vi "0 - Shooting v2.vi"(8 "Shoot Override":dbl, 9 "Serializer Override":dbl, 11 "Lock PWM":bool) -> (0 "Serializer Output":dbl, 1 "Feeder Output":dbl, 2 "Shooter PWM":dbl, 3 "Rotation Out":dbl)   [LabVIEW 2016]
uses:
  <vilib>/Rock Robotics/Network Tables/NT Read Numeric Array.vi
  <vilib>/Rock Robotics/Network Tables/NT Read Number.vi
  Robot Global Data.vi
  <vilib>/addons/control/pid/pid.llb/PID (DBL).vi
  <vilib>/addons/control/pid/NI_PID_pid.lvlib
panel:
  out "PWM Output":dbl(graph)
  in  "PID gains":T1={"proportional gain (Kc)"=0.052, "integral time (Ti, min)"=0.0, "derivative time (Td, min)"=0.002} {"derivative time (Td, min)" format="%.3f"; "integral time (Ti, min)" format="%.3f"; "proportional gain (Kc)" format="%.3f"}
  out "Aim Offset":dbl=5.0 format="%#_13g"
  out "Ball In?":i16(graph)
  out "Image width":dbl(graph)
  out "Object Width":dbl=21.666666666666668
  in  "Shooting Range":dbl=3.1 format="%#_13g"
  in  "Stop Range":dbl=0.1 format="%#_13g"
  in  "Enable PID":bool
  # "Does nothing, only used as a template for the incoming values from DB"
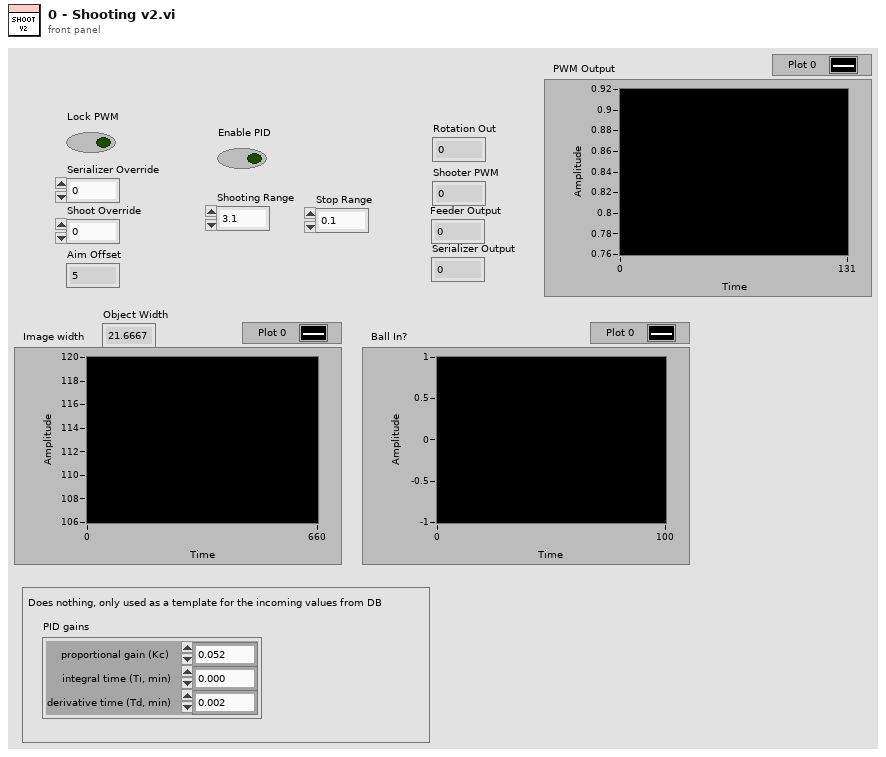
[diagram p1: front panel]
types:
  T1 = cluster{"proportional gain (Kc)":dbl, "integral time (Ti, min)":dbl, "derivative time (Td, min)":dbl}
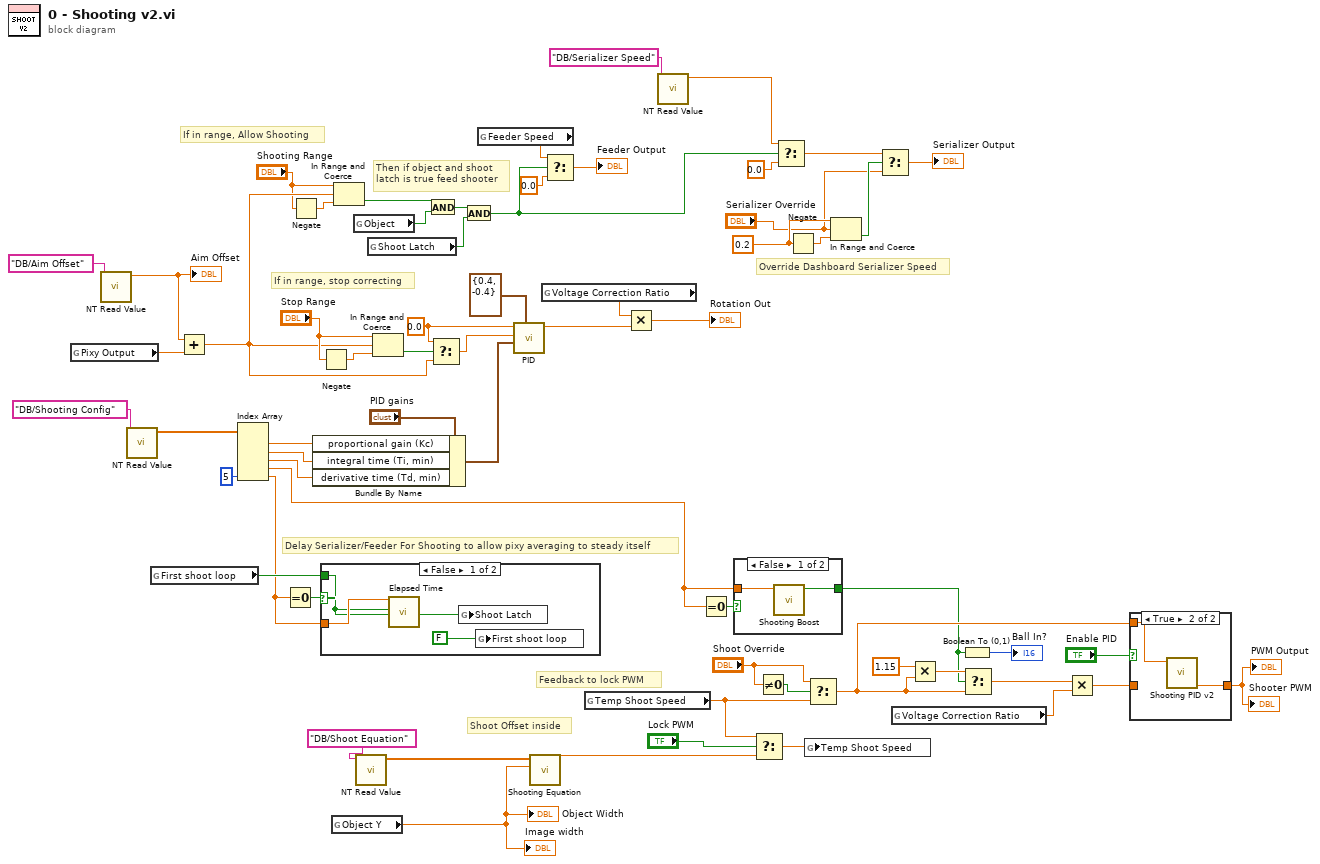
[diagram p0: block diagram]
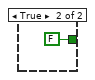
[diagram p2: hidden frame]
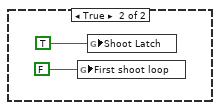
[diagram p4: hidden frame]
diagram:
  w30 = 0.2
  w44 = 0.0 ("t")
  # "Feedback to lock PWM"
  # "Override Dashboard Serializer Speed"
  # "Delay Serializer/Feeder For Shooting to allow pixy averaging to steady itself"
  # "Then if object and shoot \nlatch is true feed shooter"
  # "If in range, Allow Shooting"
  # "If in range, stop correcting"
  # "Shoot Offset inside"
  n1 = global read "Robot Global Data.vi" "Pixy Output"() -> (w49:dbl)
  n2 = call-poly <vilib>:"NT Read Value.vi"("Name"="DB/Aim Offset") -> ("Numeric"=w48:dbl)  [unwired: 9 in, 1 out]
  "Aim Offset" <- w48
  n3 = call-poly <vilib>:"NT Read Value.vi"("Name"="DB/Shooting Config") -> ("Numeric Array"=w17:dbl[])  [unwired: 9 in, 1 out]
  n4 = global read "Robot Global Data.vi" "First shoot loop"() -> (w10:bool)
  n5 = Add(x=w48, y=w49) -> (x+y=w38:dbl)
  n6 = Index Array(array=w17, index #5=5 ("index")) -> (element #1=w15:dbl, element #2=w14:dbl, element #3=w13:dbl, element #4=w1:dbl, element #5=w9:dbl)  [unwired: 4 in]
  n7 = Equal To 0?(x=w9) -> (x = 0?=w11:bool)
  n8 = Negate(x="Shooting Range") -> (-x=w37:dbl)
  n9 = Bundle By Name(cluster="PID gains", "proportional gain (Kc)"=w15, "integral time (Ti, min)"=w14, "derivative time (Td, min)"=w13) -> (w12:T1)
  n10 = Negate(x="Stop Range") -> (-x=w47:dbl)
  n11 = case shown="False" w11 {
    tunnel: w9 -> [w68 _]
    tunnel: w10 -> [w65 _]
    frame False {
      n12 = call "Elapsed Time"("Time Target (s)"=w68, "Reset"=w65, "Auto Reset"=w65) -> ("Time has Elapsed"=w67:bool)  [unwired: 9 in, 7 out]
      n13 = global write "Robot Global Data.vi" "Shoot Latch"(w67) -> ()
      n14 = global write "Robot Global Data.vi" "First shoot loop"(FALSE ("Time has Elapsed")) -> ()
    }
    frame True {
      n15 = global write "Robot Global Data.vi" "First shoot loop"(FALSE ("Time has Elapsed")) -> ()
      n16 = global write "Robot Global Data.vi" "Shoot Latch"(TRUE ("Time has Elapsed")) -> ()
    }
  }
  n17 = global read "Robot Global Data.vi" "Object Y"() -> (w62:dbl)
  "Object Width" <- w62
  "Image width" <- w62
  n18 = In Range and Coerce(upper limit="Shooting Range", x=w38, lower limit=w37) -> (In Range?=w35:bool)  [unwired: 1 out]
  n19 = global read "Robot Global Data.vi" "Object"() -> (w33:bool)
  n20 = call-poly <vilib>:"NT Read Value.vi"("Name"="DB/Shoot Equation") -> ("Numeric Array"=w63:dbl[])  [unwired: 9 in, 1 out]
  n21 = global read "Robot Global Data.vi" "Shoot Latch"() -> (w32:bool)
  n22 = In Range and Coerce(upper limit="Stop Range", x=w38, lower limit=w47) -> (In Range?=w45:bool)  [unwired: 1 out]
  n23 = And(x=w35, y=w33) -> (x .and. y?=w34:bool)
  n24 = Select(t=w44, s=w45, f=w38) -> (s? t:f=w39:dbl)
  n25 = And(x=w34, y=w32) -> (x .and. y?=w23:bool)
  n26 = global read "Robot Global Data.vi" "Feeder Speed"() -> (w26:dbl)
  n27 = call-poly <vilib>:"PID.vi"("output range"=cluster{"output high":dbl, "output low":dbl} {"output high"=0.4, "output low"=-0.4}, "PID gains"=w12, "process variable"=w39, "setpoint"=w44) -> ("output"=w41:dbl)  [unwired: 6 in, 1 out]
  n28 = call "Shooting Equation.vi"("Object Y"=w62, "Shoot Equation Parameter Array"=w63) -> ("Output"=w61:dbl)  [unwired: 9 in]
  n29 = global read "Robot Global Data.vi" "Voltage Correction Ratio"() -> (w42:dbl)
  n30 = Select(t=w26, s=w23, f=0.0) -> (s? t:f=→"Feeder Output":dbl)
  n31 = global read "Robot Global Data.vi" "Temp Shoot Speed"() -> (w58:dbl)
  n32 = Multiply(x=w42, y=w41) -> (x*y=→"Rotation Out":dbl)
  n33 = call-poly <vilib>:"NT Read Value.vi"("Name"="DB/Serializer Speed") -> ("Numeric"=w25:dbl)  [unwired: 9 in, 1 out]
  n34 = Equal To 0?(x=w1) -> (x = 0?=w3:bool)
  n35 = case shown="False" w3 {
    tunnel: [w72 FALSE ("Boost PWM")] -> w2
    tunnel: w1 -> [w71 _]
    frame False {
      n36 = call "Shooting Boost.vi"("Duration"=w71) -> ("Boost PWM"=w72:bool)  [unwired: 10 in]
    }
    frame True {
    }
  }
  n37 = Select(t=w58, s="Lock PWM", f=w61) -> (s? t:f=w59:dbl)
  n38 = Not Equal To 0?(x="Shoot Override") -> (x != 0?=w57:bool)
  n39 = Select(t=w25, s=w23, f=0.0) -> (s? t:f=w22:dbl)
  n40 = Negate(x=w30) -> (-x=w31:dbl)
  n41 = global write "Robot Global Data.vi" "Temp Shoot Speed"(w59) -> ()
  n42 = Select(t="Shoot Override", s=w57, f=w58) -> (s? t:f=w4:dbl)
  n43 = In Range and Coerce(upper limit=w30, x="Serializer Override", lower limit=w31) -> (In Range?=w21:bool)  [unwired: 1 out]
  n44 = Select(t=w22, s=w21, f="Serializer Override") -> (s? t:f=→"Serializer Output":dbl)
  n45 = global read "Robot Global Data.vi" "Voltage Correction Ratio"() -> (w51:dbl)
  n46 = Multiply(x=1.15 ("t"), y=w4) -> (x*y=w53:dbl)
  n47 = Boolean To (0,1)(Boolean=w2) -> (0, 1=→"Ball In?":i16)
  n48 = Select(t=w53, s=w2, f=w4) -> (s? t:f=w52:dbl)
  n49 = Multiply(x=w52, y=w51) -> (x*y=w5:dbl)
  n50 = case shown="True" "Enable PID" {
    tunnel: [w74 w76] -> w6
    tunnel: w5 -> [w74 _]
    tunnel: w4 -> [_ w75]
    frame False {
    }
    frame True {
      n51 = call "Shooting PID v2.vi"("Setpoint"=w75) -> ("Output"=w76:dbl)  [unwired: 10 in]
    }
  }
  "Shooter PWM" <- w6
  "PWM Output" <- w6
